vi "SIne Wave Generator_demoinfocom.vi"(8 "Phase in deg":dbl, 9 "Sampling rate":dbl format="%#_13g", 10 "Frequency":dbl format="%#_13g", 11 "Duration":dbl format="%#_13g") -> (2 "output cluster":cluster{dbl, dbl, dbl[]}, 3 "Array":dbl[](array[numeric]))   [LabVIEW 2021]
uses:
  <vilib>/Analysis/1siggen.llb/Ramp Pattern by Samples.vi
  <vilib>/Analysis/NI_AALBase.lvlib
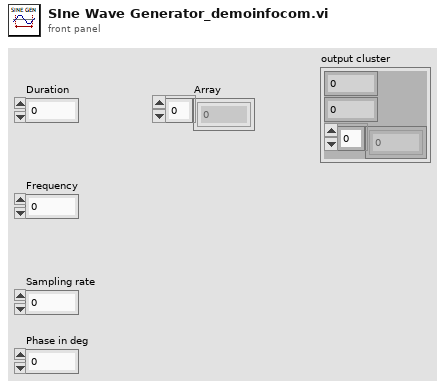
[diagram p1: front panel]
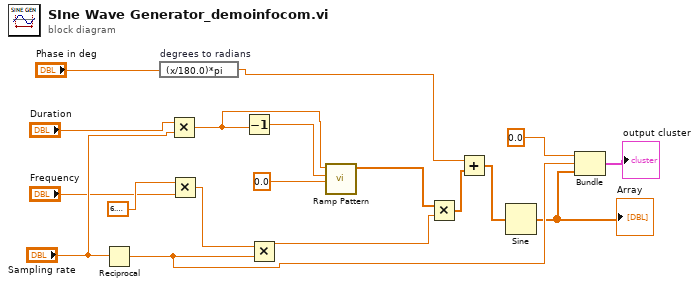
[diagram p0: block diagram]
diagram:
  n1 = Reciprocal(x="Sampling rate") -> (1/x=w7:dbl)
  n2 = expression code="(x/180.0)*pi" "degrees to radians"("Phase in deg") -> (w3:dbl)
  n3 = Multiply(x="Duration", y="Sampling rate") -> (x*y=w15:dbl)
  n4 = Multiply(x=6.283185307179586, y="Frequency") -> (x*y=w12:dbl)
  n5 = Decrement(x=w15) -> (x-1=w14:dbl)
  n6 = Multiply(x=w12, y=w7) -> (x*y=w18:dbl)
  n7 = call-poly <vilib>:"Ramp Pattern.vi"("start"=0.0, "end"=w14, "samples"=w15) -> ("Ramp Pattern"=w17:dbl[])  [unwired: 7 in, 1 out]
  n8 = Multiply(x=w17, y=w18) -> (x*y=w2:dbl[])
  n9 = Add(x=w3, y=w2) -> (x+y=w1:dbl[])
  n10 = Sine(x=w1) -> (sin(x)=w6:dbl[])
  "Array" <- w6
  n11 = Bundle(0.0, w7, w6) -> (→"output cluster":cluster{dbl, dbl, dbl[]})  [unwired: 1 in]
